vi "New Protected Subpanel.vi"(10 "SubPnl Refnum":refnum<vi>) -> (3 "Protected Subpanel":T1)   [LabVIEW 2015, in "IViewable.lvlib" / "ProtectedSubpanel.lvclass"]
uses:
  ProtectedSubpanel.lvclass
  Protected Subpanel Reference.ctl
  ProtectedSubpanel.lvclass/ProtectedSubpanel.ctl
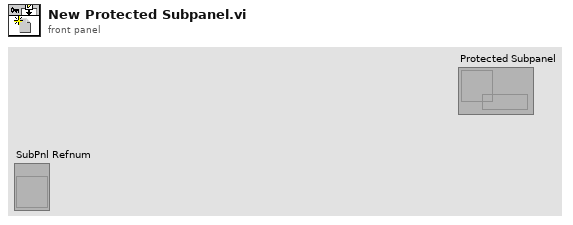
[diagram p1: front panel]
types:
  T1 = typedef "IViewable.lvlib/ProtectedSubpanel.lvclass/Protected Subpanel Reference.ctl" = refnum<data-value>
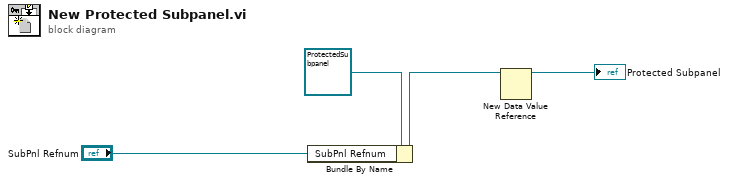
[diagram p0: block diagram]
diagram:
  n1 = Bundle By Name(cluster=refnum<class "ProtectedSubpanel.lvclass"> refnum ("ProtectedSubpanel in"), "SubPnl Refnum"="SubPnl Refnum") -> (w2:refnum<class "ProtectedSubpanel.lvclass">)
  n2 = New Data Value Reference(data value=w2) -> (data value reference=→"Protected Subpanel":refnum<data-value>)  [unwired: 1 in, 1 out]
